vi "image display handler.vi"   [LabVIEW 2012]
uses:
  Custom Controls/MAIN Image panel tab Control type def.ctl
  GFG/GFGImageRefsGet.vi
  GFG/GFG library.lvlib
types:
  T1 = typedef "MAIN Image panel tab Control type def.ctl" = enum32{"Channel 1", "Channel 2", "Channel 3", "Channel 4", "all channels", "RGB overlay", "ROI", "arbitrary line scan"}
  T2 = typedef "Image Type" = u32
  T3 = typedef "IMAQ Image.ctl" = refnum<image>
  T4 = cluster{"Channel 1 small":T3, "Channel 2 small":T3, "Channel 3 small":T3, "Channel 4 small":T3, "Channel 1 large":T3, "Channel 2 large":T3, "Channel 3 large":T3, "Channel 4 large":T3, "RGB overlay":T3, "ROI Image display":T3, "arb line scan display":T3, "Channel 5 large":T3}
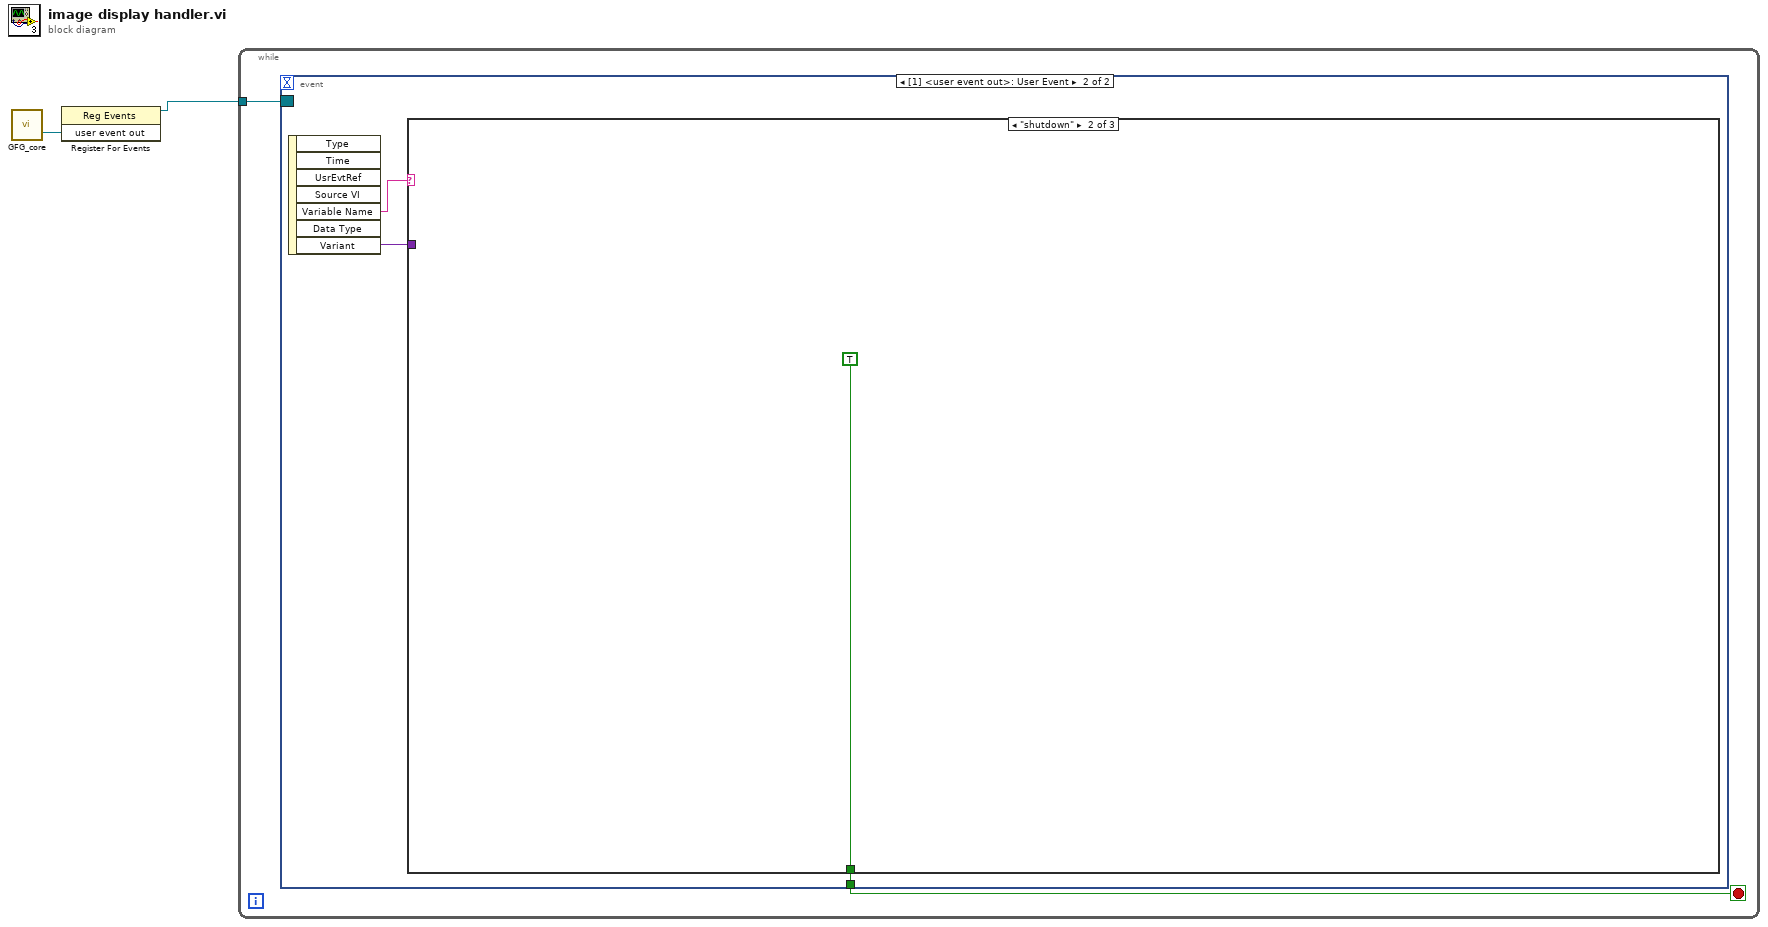
[diagram p0: block diagram]
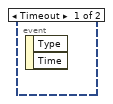
[diagram p2: hidden frame]
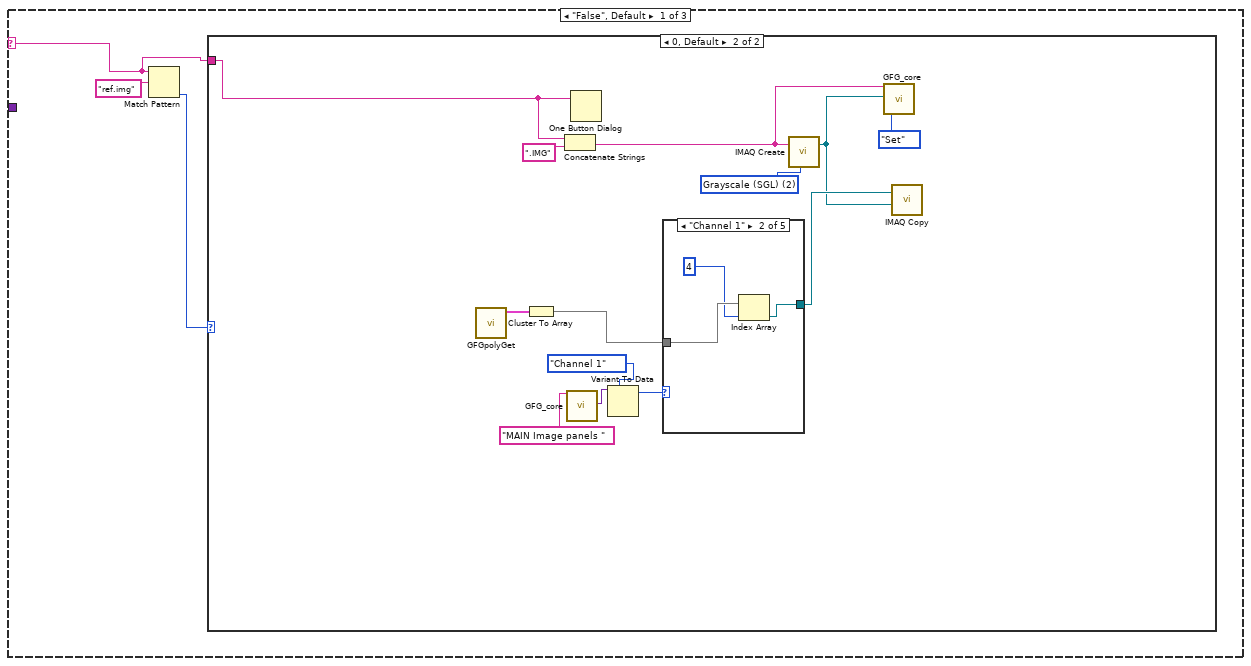
[diagram p3: hidden frame]
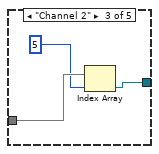
[diagram p6: hidden frame]
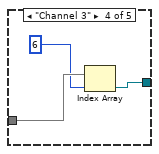
[diagram p7: hidden frame]
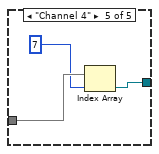
[diagram p8: hidden frame]
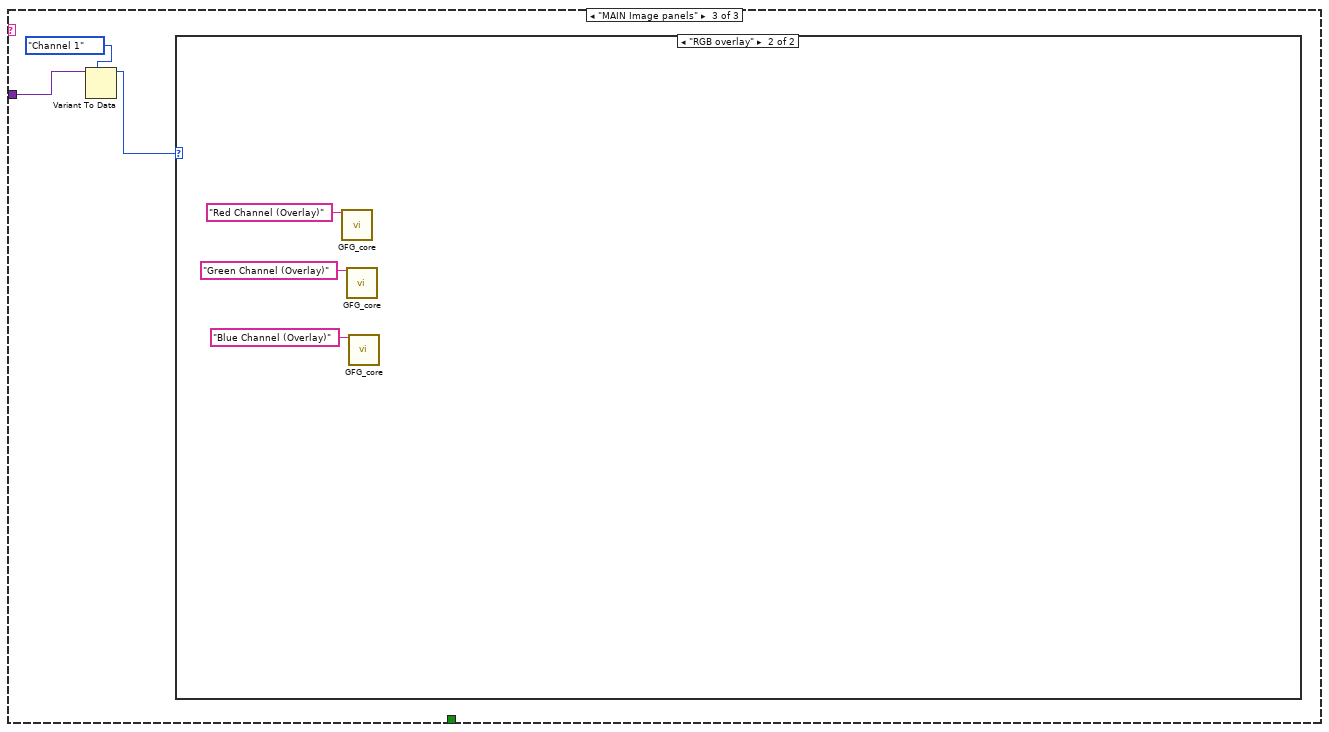
[diagram p9: hidden frame]
diagram:
  n1 = call "GFG_core.vi"() -> ("user event out"=w2:refnum<user-event>)  [unwired: 13 in, 6 out]
  n2 = register-events(w2) -> (reference out=w1:refnum<event-registration>)  [unwired: 2 in, 1 out]
  n3 = while {
    tunnel: w1 -> [w4]
    stop <- w3 stop-if-true
    n4 = event shown="[1] <user event out>: User Event" {
      selector: w4 -> [_ _]
      dyn-events: _ -> [_ _]
      timeout: _ -> [_ _]
      tunnel: [_ w6] -> w3
      event Timeout {
        n5 = event-data() -> ()  [unwired: 1 in, 2 out]
      }
      event User Event {
        n6 = event-data() -> ("Variable Name"=w7:string, "Variant"=w5:variant)  [unwired: 1 in, 5 out]
        n7 = case shown="\"shutdown\"" w7 {
          selector: w7 -> [w8 _ _]
          tunnel: [_ TRUE _] -> w6
          tunnel: w5 -> [_ _ w38]
          frame "False", Default {
            n8 = Match Pattern(string=w8, regular expression="ref.img") -> (offset past match=w9:i32)  [unwired: 1 in, 3 out]
            n9 = case shown="0, Default" w9 {
              tunnel: w8 -> [_ w17]
              frame -1 {
              }
              frame 0, Default {
                w15 = T2 2 items=["Grayscale (U8)", "Grayscale (I16)", "Grayscale (SGL)", "Complex (CSG)", "RGB (U32)", "HSL (U32)", "RGB (U64)", "Grayscale (U16)"] ("Image Type")
                n10 = call-poly "GFGpolyGet.vi"() -> ("Image Refs Out"=w19:T4)  [unwired: 10 in, 1 out]
                n11 = Cluster To Array(cluster=w19) -> (array=w18:T3[])
                n12 = Concatenate Strings(w17, ".IMG" ("string")) -> (w12:string)
                n13 = call "GFG_core.vi"("Variable Name in"="MAIN Image panels ") -> ("Variant Out"=w23:variant)  [unwired: 12 in, 6 out]
                n14 = One Button Dialog(message=w17) -> ()  [unwired: 1 in, 1 out]
                n15 = Variant To Data(type=MAIN_Image_panel_tab_Control_type_def."Channel 1" ("MAIN Image panels"), Variant=w23) -> (data=w21:T1)  [unwired: 1 in, 1 out]
                n16 = case shown="\"Channel 1\"" w21 {
                  tunnel: w18 -> [_ w26 w29 w32 w35]
                  tunnel: [_ w24 w27 w30 w33] -> w14
                  frame Default {
                  }
                  frame "Channel 1" {
                    n17 = Index Array(array=w26, index=4) -> (element=w24:T3)
                  }
                  frame "Channel 2" {
                    n18 = Index Array(array=w29, index=5) -> (element=w27:T3)
                  }
                  frame "Channel 3" {
                    n19 = Index Array(array=w32, index=6) -> (element=w30:T3)
                  }
                  frame "Channel 4" {
                    n20 = Index Array(array=w35, index=7) -> (element=w33:T3)
                  }
                }
                n21 = call "IMAQ Create"("Image Name"=w12, "Image Type"=w15) -> ("New Image"=w11:T3)  [unwired: 3 in, 1 out]
                n22 = call "GFG_core.vi"("Variable Name in"=w12, "Variant in"=w11, "Action"=enum16{"Init", "Set", "Get"}."Set") -> ()  [unwired: 10 in, 7 out]
                n23 = call "IMAQ Copy"("Image Dst"=w11, "Image Src"=w14) -> ()  [unwired: 4 in, 2 out]
              }
            }
          }
          frame "shutdown" {
          }
          frame "MAIN Image panels" {
            n24 = Variant To Data(type=MAIN_Image_panel_tab_Control_type_def."Channel 1" ("MAIN Image panels"), Variant=w38) -> (data=w37:T1)  [unwired: 1 in, 1 out]
            n25 = case shown="\"RGB overlay\"" w37 {
              frame "Channel 1", Default {
              }
              frame "RGB overlay" {
                n26 = call "GFG_core.vi"("Variable Name in"="Red Channel (Overlay)") -> ()  [unwired: 12 in, 7 out]
                n27 = call "GFG_core.vi"("Variable Name in"="Green Channel (Overlay)") -> ()  [unwired: 12 in, 7 out]
                n28 = call "GFG_core.vi"("Variable Name in"="Blue Channel (Overlay)") -> ()  [unwired: 12 in, 7 out]
              }
            }
          }
        }
      }
    }
  }
